vi "Begin.vi"() -> (0 "error out":errorcluster)   [LabVIEW 2013]
doc: "Called before other user functions, this VI is expected to open initial I/O refnums, load in file data, and do all program initialization. Notice that the <B>error out</B> terminal is simply used for data flow. Wiring it to other structures or subVIs ensures that this VI runs first."
uses:
  <vilib>/Rock Robotics/WPI/Joystick/WPI_JoystickDeviceEnum.ctl
  <vilib>/Rock Robotics/SystemInterfaces/Typedef/FPGA_TypedefDigitalModule.ctl
  <vilib>/Rock Robotics/SystemInterfaces/DIO/FPGA_DIOChannel.ctl
  <vilib>/Rock Robotics/SystemInterfaces/DIO/FPGA_DIORelayChannel.ctl
  <vilib>/Rock Robotics/SystemInterfaces/Typedef/FPGA_TypedefSolenoidModule.ctl
  <vilib>/Rock Robotics/WPI/Solenoid/WPI_SolenoidChannel.ctl
  <vilib>/Rock Robotics/WPI/Solenoid/WPI_SolenoidValue.ctl
  <vilib>/Rock Robotics/SystemInterfaces/DIO/FPGA_DIOPWMChannel.ctl
  <vilib>/Rock Robotics/WPI/Encoder/WPI_EncoderType.ctl
  <vilib>/Rock Robotics/WPI/Solenoid/WPI_SolenoidOpenDouble.vi
  <vilib>/Rock Robotics/WPI/Solenoid/WPI_SolenoidSetEnum.vi
  <vilib>/Rock Robotics/WPI/Counter/WPI_CounterDigitalInputToDigitalSource.vi
  <vilib>/Rock Robotics/WPI/RobotDrive/WPI_RobotDriveOpen2MotorWithVictor.vi
  <vilib>/Rock Robotics/WPI/MotorControl/WPI_MotorControlOpen Victor.vi
  <vilib>/Rock Robotics/WPI/Compressor/WPI_CompressorGetSetRefNum.vi
  <vilib>/Rock Robotics/WPI/Camera/WPI_CameraImageSize.ctl
  <vilib>/Rock Robotics/WPI/Camera/WPI_CameraWhite Balance Values.ctl
  <vilib>/Rock Robotics/WPI/Camera/WPI_CameraExposure Values.ctl
  <vilib>/Rock Robotics/WPI/Camera/WPI_CameraFrameRate.ctl
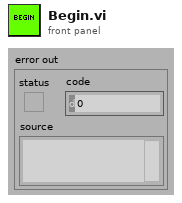
[diagram p1: front panel]
types:
  T1 = typedef "FPGA_DIOChannel.ctl" = enum8{"DIO 1", "DIO 2", "DIO 3", "DIO 4", "DIO 5", "DIO 6", "DIO 7", "DIO 8", "DIO 9", "DIO 10", "DIO 11", "DIO 12", "DIO 13", "DIO 14", "Invalid"}
  T2 = typedef "WPI_SolenoidChannel.ctl" = enum8{"Solenoid 1", "Solenoid 2", "Solenoid 3", "Solenoid 4", "Solenoid 5", "Solenoid 6", "Solenoid 7", "Solenoid 8", "Invalid"}
  T3 = typedef "FPGA_DIOPWMChannel.ctl" = enum8{"PWM 1", "PWM 2", "PWM 3", "PWM 4", "PWM 5", "PWM 6", "PWM 7", "PWM 8", "PWM 9", "PWM 10", "Invalid"}
  T4 = typedef "WPI_EncoderType.ctl" = enum16{"1x", "2x", "4x"}
  T5 = typedef "WPI_SolenoidValue.ctl" = enum16{"Off", "On", "Forward", "Reverse"}
  T6 = typedef "FPGA_TypedefSolenoidModule.ctl" = enum16{"Solenoid Module 1", "Solenoid Module 2"}
  T7 = typedef "FPGA_DIORelayChannel.ctl" = enum8{"Relay 1", "Relay 2", "Relay 3", "Relay 4", "Relay 5", "Relay 6", "Relay 7", "Relay 8", "Invalid"}
  T8 = typedef "WPI_JoystickDeviceEnum.ctl" = enum16{"USB 1", "USB 2", "USB 3", "USB 4", "Kinect 1", "Kinect 2"}
  T9 = typedef "FPGA_TypedefDigitalModule.ctl" = enum16{"Digital Module 1", "Digital Module 2"}
  T10 = typedef "WPI_CameraFrameRate.ctl" = u32
  T11 = typedef "WPI_CameraExposure Values.ctl" = enum16{"Auto", "Flicker-free 50 Hz", "Flicker-free 60 Hz", "Hold current"}
  T12 = typedef "WPI_CameraWhite Balance Values.ctl" = enum16{"Auto", "Fixed indoor", "Fixed outdoor 1", "Fixed outdoor 2", "Fixed fluorescent 1", "Fixed fluorescent 2", "Hold current"}
  T13 = typedef "WPI_CameraImageSize.ctl" = enum16{"640x480", "320x240", "160x120"}
  T14 = typedef "WPI_CameraDevRef.ctl" = cluster{"Camera Address":string, "CameraStatus":errorcluster, "Acquire Image Notifier":refnum<notifier>}
  T15 = typedef "WPI_DigitalInputDevRef.ctl" = cluster{"DevStatus":errorcluster, "DIO Channel":T1, "Digital Module":T9}
  T16 = typedef "WPI_MotorControlDeviceRef.ctl" = cluster{"DeviceStatus":errorcluster, "Type":enum16{"PWM", "CAN"}, "PWM":cluster{"Digital Module":T9, "PWM Channel":T3, "DeadBand":T17}, "CAN":cluster{"Device Number":u8, "Control Mode":T18, "Semaphore":T19, "Max Vout":dbl}, "Invert":bool, "TransformRef":T20, "InvTransformRef":T20}
  T17 = typedef "WPI_PWMDeadband.ctl" = cluster{"Name":string, "maxPositivePwm":i32, "minPositivePwm":i32, "centerPwm":i32, "maxNegativePwm":i32, "minNegativePwm":i32, "angularRange":u16}
  T18 = typedef "WPI_CANJaguar_ControlMode.ctl" = enum8{"Percent VBus", "Current", "Speed", "Position", "Voltage"}
  T19 = typedef "Semaphore RefNum" = refnum<k1>
  T20 = typedef "WPI_PWMTransform_ConPane.ctl" = refnum<vi>
  T21 = typedef "WPI_SolenoidDevRef.ctl" = cluster{"DevStatus":errorcluster, "Solenoid Module":T6, "Forward Solenoid Channel":T2, "Reverse Solenoid Channel":T2}
  T22 = typedef "FPGA_CounterEncoderSourceConvertionLVSourceType.ctl" = cluster{"DevStatus":errorcluster, "AnalogTriggerMode?":bool, "DigitalMode":cluster{"Digital Module":T9, "DIO Channel":T23}, "AnalogTriggerMode":cluster{"AnalogTriggerIndex":T24, "OutputType":T25}}
  T23 = typedef "FPGA_DIODigitalSourceChannel.ctl" = enum8{"DIO 1", "DIO 2", "DIO 3", "DIO 4", "DIO 5", "DIO 6", "DIO 7", "DIO 8", "DIO 9", "DIO 10", "DIO 11", "DIO 12", "DIO 13", "DIO 14", "Disabled"}
  T24 = typedef "FPGA_AnalogTriggerIndex.ctl" = enum8{"Trig 0", "Trig 1", "Trig 2", "Trig 3", "Trig 4", "Trig 5", "Trig 6", "Trig 7", "Invalid"}
  T25 = typedef "FPGA_AnalogTriggerOutType.ctl" = enum16{"InWindow", "TriggerState", "Rising", "Falling"}
  T26 = typedef "WPI_CompressorDevRef.ctl" = cluster{"DevStatus":errorcluster, "DigitalInputDevRef":T15, "RelayDevRef":T27}
  T27 = typedef "WPI_RelayDevRef.ctl" = cluster{"DevStatus":errorcluster, "Relay Channel":T7, "Digital Module":T9, "Relay Direction":T28}
  T28 = typedef "WPI_RelayDirection.ctl" = enum16{"Both directions", "Forward only", "Reverse only"}
  T29 = typedef "WPI_RobotDriveDevRef.ctl" = cluster{"DevStatus":errorcluster, "Motors[]":T16[], "Square Inputs":bool, "Max Output":dbl, "Isochronous":bool}
  T30 = typedef "WPI_EncoderDevRef.ctl" = cluster{"DevStatus":errorcluster, "EncoderIndex":T31, "CounterIndex":T32, "DistancePerCount":dbl, "Decoding Type":T4}
  T31 = typedef "FPGA_EncoderIdx.ctl" = enum8{"Enc 0", "Enc 1", "Enc 2", "Enc 3", "Invalid"}
  T32 = typedef "FPGA_CounterCtrSystemIndex.ctl" = enum8{"Ctr 0", "Ctr 1", "Ctr 2", "Ctr 3", "Ctr 4", "Ctr 5", "Ctr 6", "Ctr 7", "Invalid"}
  T33 = typedef "WPI_JoystickDevRef.ctl" = cluster{"Device":T8}
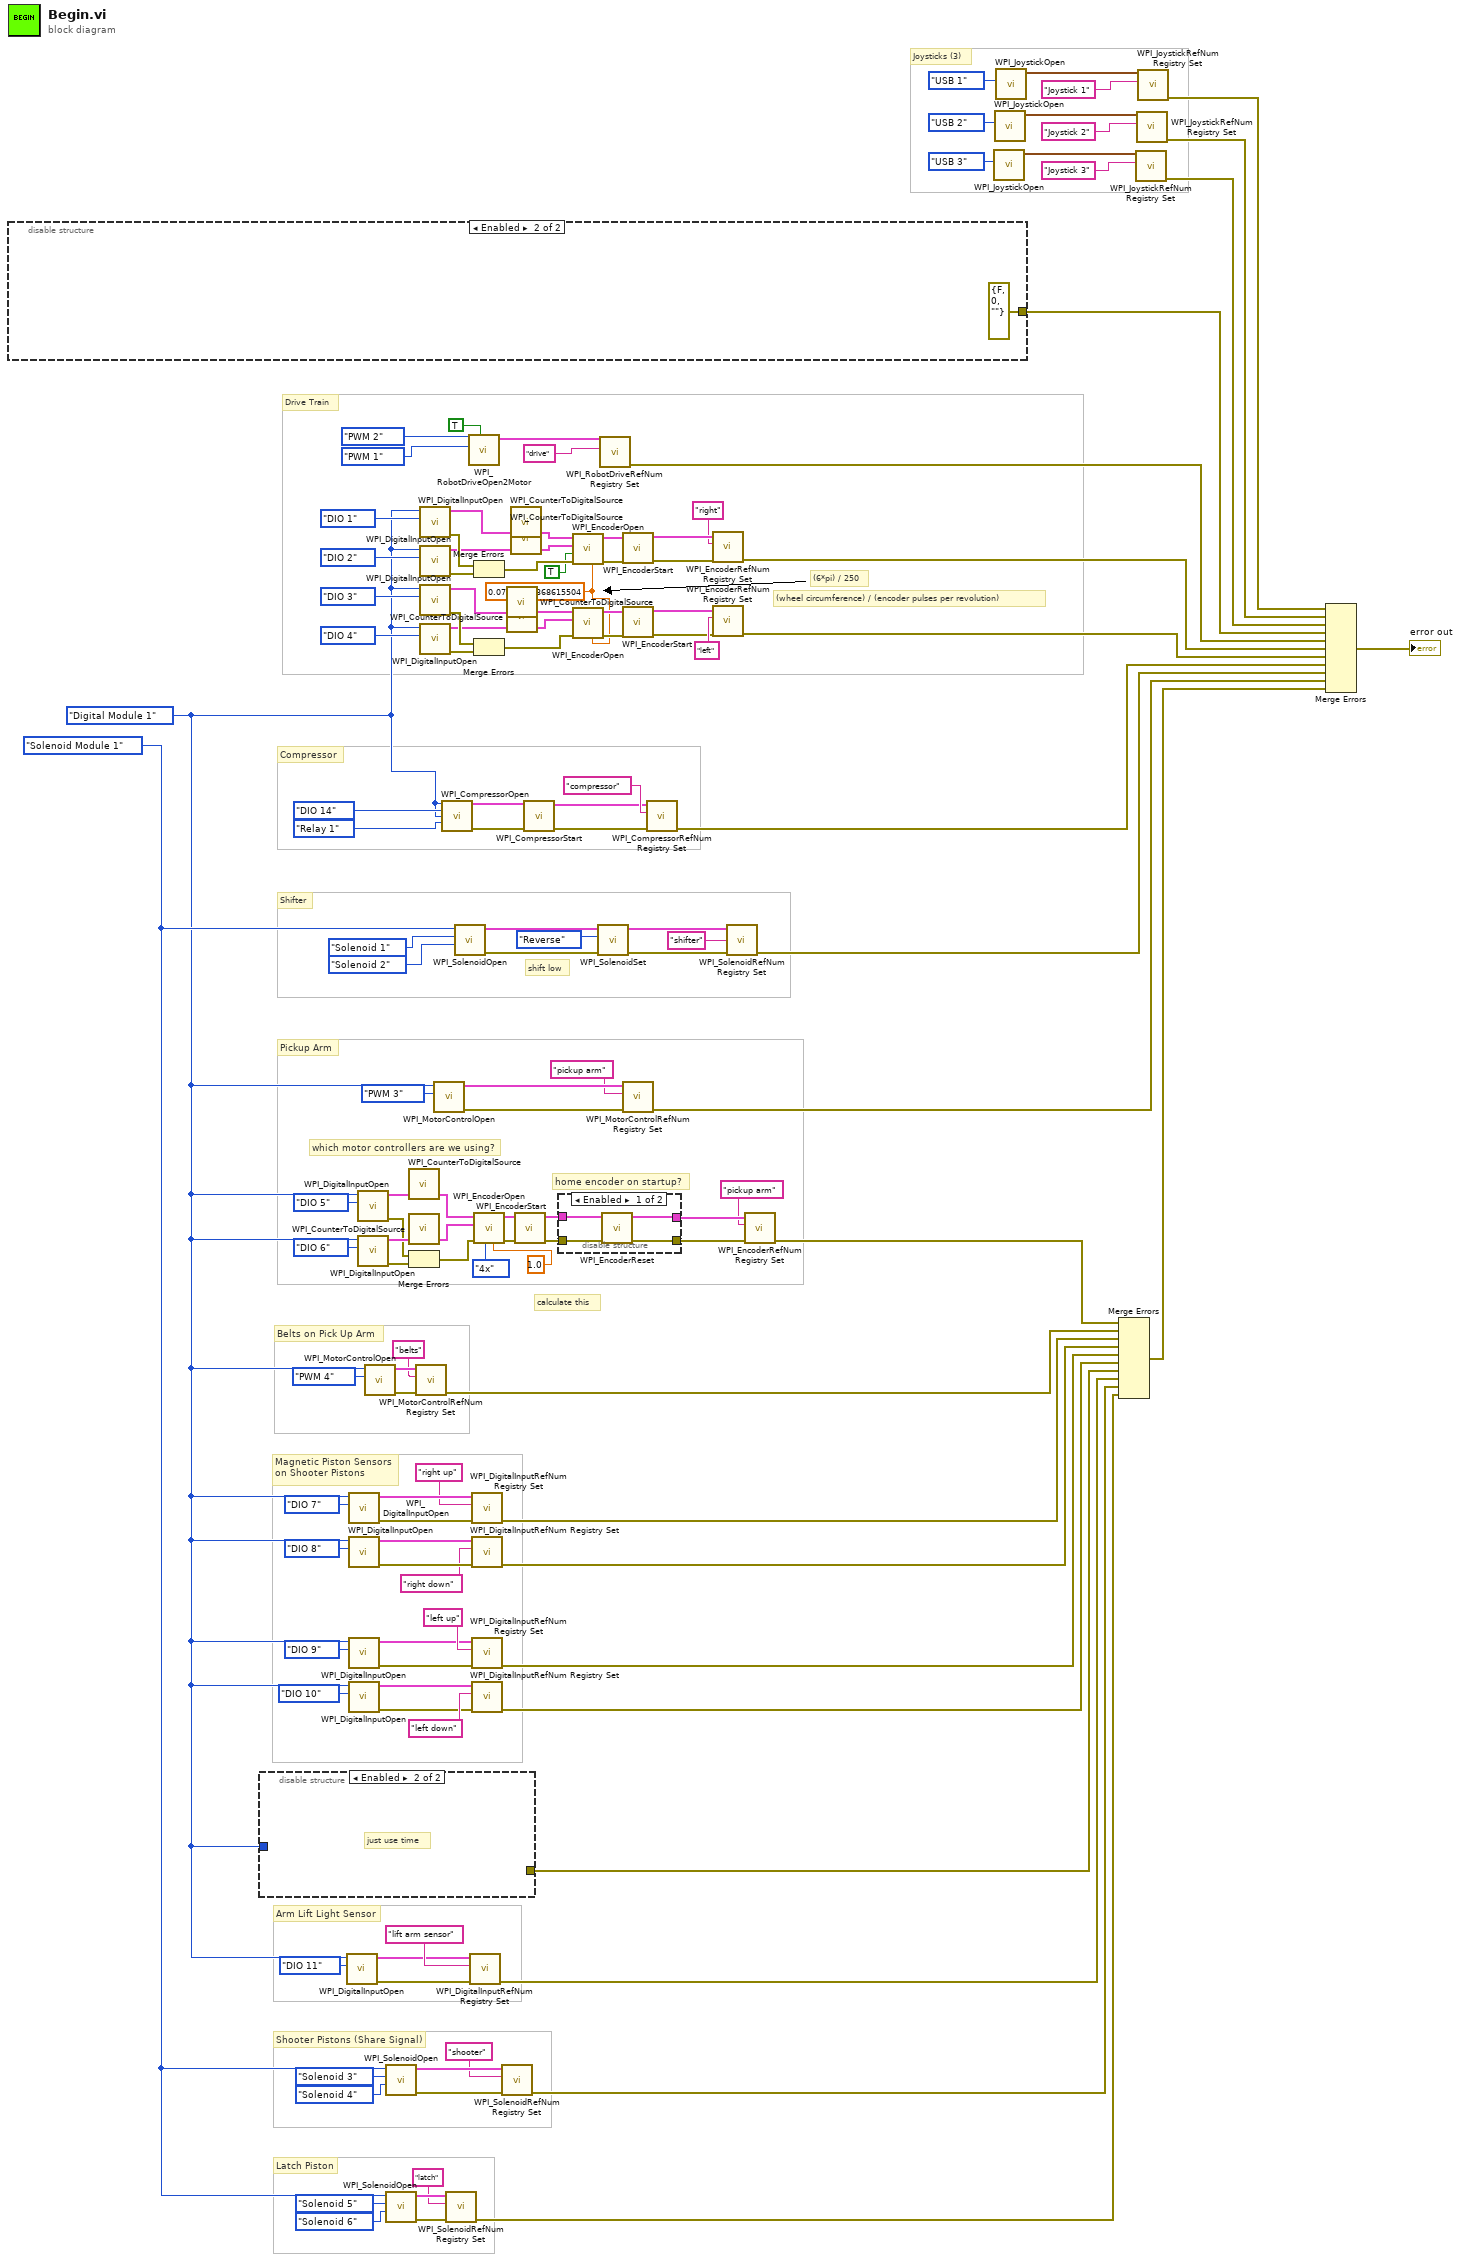
[diagram p0: block diagram]
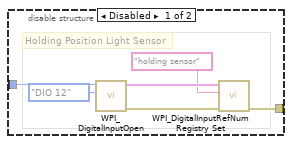
[diagram p2: hidden frame]
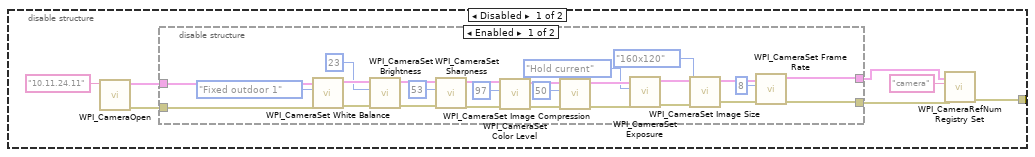
[diagram p4: hidden frame]
diagram:
  w83 = 0.07539822368615504 ("DistancePerCount")
  w20 = FPGA_TypedefSolenoidModule."Solenoid Module 1" ("Solenoid Module (Module 1)")
  w7 = FPGA_TypedefDigitalModule."Digital Module 1" ("Digital Module (Module 1)")
  # "Arm Lift Light Sensor"
  # "Joysticks (3)"
  # "Latch Piston"
  # "Shooter Pistons (Share Signal)"
  # "Magnetic Piston Sensors\non Shooter Pistons"
  # "Belts on Pick Up Arm"
  # "calculate this"
  # "Pickup Arm"
  # "home encoder on startup?"
  # "Shifter"
  # "Compressor"
  # "Drive Train"
  # "which motor controllers are we using?"
  # "shift low"
  # "(wheel circumference) / (encoder pulses per revolution)"
  # "(6*pi) / 250"
  n1 = disable-structure shown="Enabled" {
    disable-tunnel: [w140 errorcluster {"status"=FALSE, "code"=0, "source"=""} ("error out")] -> w127
    frame Disabled {
      n2 = call <vilib>:"WPI_CameraOpen.vi"("Camera Address"="10.11.24.11") -> ("error out"=w142:errorcluster, "CameraDevRef"=w144:T14)  [unwired: 9 in]
      n3 = disable-structure shown="Enabled" {
        disable-tunnel: w144 -> [w170 w174]
        disable-tunnel: [w148 w174] -> w143
        disable-tunnel: w142 -> [w157 w173]
        disable-tunnel: [w147 w173] -> w141
        frame Enabled {
          n4 = call <vilib>:"WPI_CameraSet White Balance.vi"("error in (no error)"=w157, "White Balance"=WPI_CameraWhite_Balance_Values."Fixed outdoor 1", "CameraDevRef"=w170) -> ("error out"=w158:errorcluster, "CameraDevRef Out"=w169:T14)  [unwired: 7 in]
          n5 = call <vilib>:"WPI_CameraSet Brightness.vi"("error in (no error)"=w158, "Brightness"=23, "CameraDevRef"=w169) -> ("error out"=w159:errorcluster, "CameraDevRef Out"=w168:T14)  [unwired: 7 in]
          n6 = call <vilib>:"WPI_CameraSet Sharpness.vi"("error in (no error)"=w159, "Sharpness"=53, "CameraDevRef"=w168) -> ("error out"=w160:errorcluster, "CameraDevRef Out"=w167:T14)  [unwired: 7 in]
          n7 = call <vilib>:"WPI_CameraSet Color Level.vi"("error in (no error)"=w160, "Color Level"=97, "CameraDevRef"=w167) -> ("error out"=w161:errorcluster, "CameraDevRef Out"=w166:T14)  [unwired: 7 in]
          n8 = call <vilib>:"WPI_CameraSet Image Compression.vi"("error in (no error)"=w161, "Compression"=50, "CameraDevRef"=w166) -> ("error out"=w172:errorcluster, "CameraDevRef Out"=w171:T14)  [unwired: 7 in]
          n9 = call <vilib>:"WPI_CameraSet Exposure.vi"("error in (no error)"=w172, "Exposure"=WPI_CameraExposure_Values."Hold current", "CameraDevRef"=w171) -> ("error out"=w162:errorcluster, "CameraDevRef Out"=w165:T14)  [unwired: 7 in]
          n10 = call <vilib>:"WPI_CameraSet Image Size.vi"("error in (no error)"=w162, "Image Size"=WPI_CameraImageSize."160x120", "CameraDevRef"=w165) -> ("error out"=w163:errorcluster, "CameraDevRef Out"=w164:T14)  [unwired: 7 in]
          n11 = call <vilib>:"WPI_CameraSet Frame Rate.vi"("error in (no error)"=w163, "Frame Rate (fps)"=T10 8, "CameraDevRef"=w164) -> ("error out"=w147:errorcluster, "CameraDevRef Out"=w148:T14)  [unwired: 7 in]
        }
        frame Disabled {
        }
      }
      n12 = call <vilib>:"WPI_CameraRefNum Registry Set.vi"("error in (no error)"=w141, "refnum name"="camera", "CameraDevRef"=w143) -> ("error out"=w140:errorcluster)  [unwired: 7 in, 1 out]
    }
    frame Enabled {
    }
  }
  n13 = disable-structure shown="Enabled" {
    disable-tunnel: w7 -> [w177 _]
    disable-tunnel: [w176 _] -> w3
    frame Disabled {
      # "Holding Position Light Sensor"
      n14 = call <vilib>:"WPI_DigitalInputOpen.vi"("DIO Channel"=FPGA_DIOChannel."DIO 12", "Digital Module (Module 1)"=w177) -> ("error out"=w180:errorcluster, "DigitalInputDevRef"=w179:T15)  [unwired: 8 in]
      n15 = call <vilib>:"WPI_DigitalInputRefNum Registry Set.vi"("error in (no error)"=w180, "refnum name"="holding sensor", "DigitalInputDevRef"=w179) -> ("error out"=w176:errorcluster)  [unwired: 7 in, 1 out]
    }
    frame Enabled {
      # "just use time"
    }
  }
  n16 = call <vilib>:"WPI_DigitalInputOpen.vi"("DIO Channel"=FPGA_DIOChannel."DIO 11", "Digital Module (Module 1)"=w7) -> ("error out"=w17:errorcluster, "DigitalInputDevRef"=w18:T15)  [unwired: 8 in]
  n17 = call <vilib>:"WPI_DigitalInputOpen.vi"("DIO Channel"=FPGA_DIOChannel."DIO 7", "Digital Module (Module 1)"=w7) -> ("error out"=w40:errorcluster, "DigitalInputDevRef"=w39:T15)  [unwired: 8 in]
  n18 = call <vilib>:"WPI_DigitalInputOpen.vi"("DIO Channel"=FPGA_DIOChannel."DIO 8", "Digital Module (Module 1)"=w7) -> ("error out"=w38:errorcluster, "DigitalInputDevRef"=w37:T15)  [unwired: 8 in]
  n19 = call <vilib>:"WPI_DigitalInputOpen.vi"("DIO Channel"=FPGA_DIOChannel."DIO 9", "Digital Module (Module 1)"=w7) -> ("error out"=w8:errorcluster, "DigitalInputDevRef"=w9:T15)  [unwired: 8 in]
  n20 = call <vilib>:"WPI_DigitalInputOpen.vi"("DIO Channel"=FPGA_DIOChannel."DIO 10", "Digital Module (Module 1)"=w7) -> ("error out"=w10:errorcluster, "DigitalInputDevRef"=w11:T15)  [unwired: 8 in]
  n21 = call <vilib>:"WPI_DigitalInputOpen.vi"("DIO Channel"=FPGA_DIOChannel."DIO 5", "Digital Module (Module 1)"=w7) -> ("error out"=w58:errorcluster, "DigitalInputDevRef"=w63:T15)  [unwired: 8 in]
  n22 = call <vilib>:"WPI_DigitalInputOpen.vi"("DIO Channel"=FPGA_DIOChannel."DIO 6", "Digital Module (Module 1)"=w7) -> ("error out"=w59:errorcluster, "DigitalInputDevRef"=w62:T15)  [unwired: 8 in]
  n23 = call-poly <vilib>:"WPI_MotorControlOpen.vi"("PWM Channel"=FPGA_DIOPWMChannel."PWM 4", "Digital Module (Module 1)"=w7) -> ("error out"=w46:errorcluster, "MotorControlDeviceRef"=w45:T16)  [unwired: 8 in]
  n24 = call-poly <vilib>:"WPI_SolenoidOpen.vi"("Reverse Solenoid Channel"=WPI_SolenoidChannel."Solenoid 4", "Forward Solenoid Channel"=WPI_SolenoidChannel."Solenoid 3", "Solenoid Module (Module 1)"=w20) -> ("error out"=w26:errorcluster, "SolenoidDevRef"=w25:T21)  [unwired: 7 in]
  n25 = call-poly <vilib>:"WPI_SolenoidOpen.vi"("Reverse Solenoid Channel"=WPI_SolenoidChannel."Solenoid 6", "Forward Solenoid Channel"=WPI_SolenoidChannel."Solenoid 5", "Solenoid Module (Module 1)"=w20) -> ("error out"=w24:errorcluster, "SolenoidDevRef"=w23:T21)  [unwired: 7 in]
  n26 = call-poly <vilib>:"WPI_CounterToDigitalSource.vi"("DigitalInputDevRef"=w63) -> ("Digital Source"=w61:T22)  [unwired: 6 in]
  n27 = call-poly <vilib>:"WPI_CounterToDigitalSource.vi"("DigitalInputDevRef"=w62) -> ("Digital Source"=w60:T22)  [unwired: 6 in]
  n28 = Merge Errors(w58, w59) -> (w57:errorcluster)
  n29 = call <vilib>:"WPI_MotorControlRefNum Registry Set.vi"("error in (no error)"=w46, "refnum name"="belts", "MotorControlDevRef"=w45) -> ("error out"=w43:errorcluster)  [unwired: 7 in, 1 out]
  n30 = call <vilib>:"WPI_DigitalInputOpen.vi"("DIO Channel"=FPGA_DIOChannel."DIO 1", "Digital Module (Module 1)"=w7) -> ("error out"=w77:errorcluster, "DigitalInputDevRef"=w91:T15)  [unwired: 8 in]
  n31 = call <vilib>:"WPI_DigitalInputOpen.vi"("DIO Channel"=FPGA_DIOChannel."DIO 2", "Digital Module (Module 1)"=w7) -> ("error out"=w79:errorcluster, "DigitalInputDevRef"=w76:T15)  [unwired: 8 in]
  n32 = call <vilib>:"WPI_DigitalInputOpen.vi"("DIO Channel"=FPGA_DIOChannel."DIO 3", "Digital Module (Module 1)"=w7) -> ("error out"=w80:errorcluster, "DigitalInputDevRef"=w105:T15)  [unwired: 8 in]
  n33 = call <vilib>:"WPI_DigitalInputOpen.vi"("DIO Channel"=FPGA_DIOChannel."DIO 4", "Digital Module (Module 1)"=w7) -> ("error out"=w82:errorcluster, "DigitalInputDevRef"=w75:T15)  [unwired: 8 in]
  n34 = call-poly <vilib>:"WPI_MotorControlOpen.vi"("PWM Channel"=FPGA_DIOPWMChannel."PWM 3", "Digital Module (Module 1)"=w7) -> ("error out"=w70:errorcluster, "MotorControlDeviceRef"=w69:T16)  [unwired: 8 in]
  n35 = call <vilib>:"WPI_CompressorOpen.vi"("Pressure Switch Digital Module (Module 1)"=w7, "Pressure Switch DIO Channel"=FPGA_DIOChannel."DIO 14", "Relay Digital Module (Module 1)"=w7, "Relay Channel"=FPGA_DIORelayChannel."Relay 1") -> ("CompressorDevRef"=w119:T26, "error out"=w118:errorcluster)  [unwired: 10 in]
  n36 = call <vilib>:"WPI_SolenoidRefNum Registry Set.vi"("error in (no error)"=w24, "refnum name"="latch", "SolenoidDevRef"=w23) -> ("error out"=w6:errorcluster)  [unwired: 7 in, 1 out]
  n37 = call-poly <vilib>:"WPI_SolenoidOpen.vi"("Reverse Solenoid Channel"=WPI_SolenoidChannel."Solenoid 2", "Forward Solenoid Channel"=WPI_SolenoidChannel."Solenoid 1", "Solenoid Module (Module 1)"=w20) -> ("error out"=w110:errorcluster, "SolenoidDevRef"=w111:T21)  [unwired: 7 in]
  n38 = call-poly <vilib>:"WPI_RobotDriveOpen2Motor.vi"("Left Motor Inverted"=TRUE, "Right Motor"=FPGA_DIOPWMChannel."PWM 1", "Left Motor"=FPGA_DIOPWMChannel."PWM 2") -> ("RobotDriveDevRef"=w107:T29)  [unwired: 7 in, 1 out]
  n39 = call <vilib>:"WPI_DigitalInputRefNum Registry Set.vi"("error in (no error)"=w17, "refnum name"="lift arm sensor", "DigitalInputDevRef"=w18) -> ("error out"=w4:errorcluster)  [unwired: 7 in, 1 out]
  n40 = call <vilib>:"WPI_DigitalInputRefNum Registry Set.vi"("error in (no error)"=w40, "refnum name"="right up", "DigitalInputDevRef"=w39) -> ("error out"=w33:errorcluster)  [unwired: 7 in, 1 out]
  n41 = call <vilib>:"WPI_DigitalInputRefNum Registry Set.vi"("error in (no error)"=w38, "refnum name"="right down", "DigitalInputDevRef"=w37) -> ("error out"=w32:errorcluster)  [unwired: 7 in, 1 out]
  n42 = call <vilib>:"WPI_DigitalInputRefNum Registry Set.vi"("error in (no error)"=w8, "refnum name"="left up", "DigitalInputDevRef"=w9) -> ("error out"=w2:errorcluster)  [unwired: 7 in, 1 out]
  n43 = call <vilib>:"WPI_DigitalInputRefNum Registry Set.vi"("error in (no error)"=w10, "refnum name"="left down", "DigitalInputDevRef"=w11) -> ("error out"=w1:errorcluster)  [unwired: 7 in, 1 out]
  n44 = Merge Errors(w77, w79) -> (w78:errorcluster)
  n45 = Merge Errors(w80, w82) -> (w81:errorcluster)
  n46 = call <vilib>:"WPI_EncoderOpen.vi"("DistancePerCount"=1.0, "Decoding Type"=WPI_EncoderType."4x", "error in (no error)"=w57, "BSource"=w60, "ASource"=w61) -> ("error out"=w56:errorcluster, "EncoderDevRef"=w55:T30)  [unwired: 5 in]
  n47 = call <vilib>:"WPI_SolenoidRefNum Registry Set.vi"("error in (no error)"=w26, "refnum name"="shooter", "SolenoidDevRef"=w25) -> ("error out"=w5:errorcluster)  [unwired: 7 in, 1 out]
  n48 = call-poly <vilib>:"WPI_CounterToDigitalSource.vi"("DigitalInputDevRef"=w105) -> ("Digital Source"=w98:T22)  [unwired: 6 in]
  n49 = call-poly <vilib>:"WPI_CounterToDigitalSource.vi"("DigitalInputDevRef"=w75) -> ("Digital Source"=w99:T22)  [unwired: 6 in]
  n50 = call-poly <vilib>:"WPI_CounterToDigitalSource.vi"("DigitalInputDevRef"=w91) -> ("Digital Source"=w97:T22)  [unwired: 6 in]
  n51 = call-poly <vilib>:"WPI_CounterToDigitalSource.vi"("DigitalInputDevRef"=w76) -> ("Digital Source"=w96:T22)  [unwired: 6 in]
  n52 = call <vilib>:"WPI_EncoderStart.vi"("error in (no error)"=w56, "EncoderDevRef"=w55) -> ("error out"=w54:errorcluster, "EncoderDevRef"=w53:T30)  [unwired: 8 in]
  n53 = call <vilib>:"WPI_CompressorStart.vi"("error in (no error)"=w118, "CompressorDevRef"=w119) -> ("error out"=w117:errorcluster, "CompressorDevRef"=w116:T26)  [unwired: 8 in]
  n54 = disable-structure shown="Enabled" {
    disable-tunnel: w54 -> [w185 w186]
    disable-tunnel: w53 -> [w184 w187]
    disable-tunnel: [w183 w187] -> w51
    disable-tunnel: [w182 w186] -> w52
    frame Enabled {
      n55 = call <vilib>:"WPI_EncoderReset.vi"("error in (no error)"=w185, "EncoderDevRef"=w184) -> ("error out"=w182:errorcluster, "EncoderDevRef"=w183:T30)  [unwired: 8 in]
    }
    frame Disabled {
    }
  }
  n56 = call <vilib>:"WPI_EncoderOpen.vi"("DistancePerCount"=w83, "error in (no error)"=w78, "Invert Direction (False)"=TRUE, "BSource"=w96, "ASource"=w97) -> ("error out"=w95:errorcluster, "EncoderDevRef"=w94:T30)  [unwired: 5 in]
  n57 = call <vilib>:"WPI_EncoderOpen.vi"("DistancePerCount"=w83, "error in (no error)"=w81, "BSource"=w99, "ASource"=w98) -> ("error out"=w100:errorcluster, "EncoderDevRef"=w101:T30)  [unwired: 6 in]
  n58 = call-poly <vilib>:"WPI_SolenoidSet.vi"("error in (no error)"=w110, "Value"=WPI_SolenoidValue."Reverse", "SolenoidDevRef"=w111) -> ("error out"=w109:errorcluster, "SolenoidDevRef"=w108:T21)  [unwired: 7 in]
  n59 = call <vilib>:"WPI_RobotDriveRefNum Registry Set.vi"("refnum name"="drive", "RobotDriveDevRef"=w107) -> ("error out"=w126:errorcluster)  [unwired: 8 in, 1 out]
  n60 = call <vilib>:"WPI_EncoderStart.vi"("error in (no error)"=w95, "EncoderDevRef"=w94) -> ("error out"=w93:errorcluster, "EncoderDevRef"=w92:T30)  [unwired: 8 in]
  n61 = call <vilib>:"WPI_EncoderStart.vi"("error in (no error)"=w100, "EncoderDevRef"=w101) -> ("error out"=w102:errorcluster, "EncoderDevRef"=w103:T30)  [unwired: 8 in]
  n62 = call <vilib>:"WPI_MotorControlRefNum Registry Set.vi"("error in (no error)"=w70, "refnum name"="pickup arm", "MotorControlDevRef"=w69) -> ("error out"=w66:errorcluster)  [unwired: 7 in, 1 out]
  n63 = call <vilib>:"WPI_CompressorRefNum Registry Set.vi"("error in (no error)"=w117, "refnum name"="compressor", "CompressorDevRef"=w116) -> ("error out"=w71:errorcluster)  [unwired: 7 in, 1 out]
  n64 = call <vilib>:"WPI_EncoderRefNum Registry Set.vi"("error in (no error)"=w93, "refnum name"="right", "EncoderDevRef"=w92) -> ("error out"=w125:errorcluster)  [unwired: 7 in, 1 out]
  n65 = call <vilib>:"WPI_EncoderRefNum Registry Set.vi"("error in (no error)"=w102, "refnum name"="left", "EncoderDevRef"=w103) -> ("error out"=w124:errorcluster)  [unwired: 7 in, 1 out]
  n66 = call <vilib>:"WPI_SolenoidRefNum Registry Set.vi"("error in (no error)"=w109, "refnum name"="shifter", "SolenoidDevRef"=w108) -> ("error out"=w72:errorcluster)  [unwired: 7 in, 1 out]
  n67 = call <vilib>:"WPI_EncoderRefNum Registry Set.vi"("error in (no error)"=w52, "refnum name"="pickup arm", "EncoderDevRef"=w51) -> ("error out"=w42:errorcluster)  [unwired: 7 in, 1 out]
  n68 = call <vilib>:"WPI_JoystickOpen.vi"("JoystickDevice"=WPI_JoystickDeviceEnum."USB 3") -> ("JoystickDevRef"=w138:T33)  [unwired: 10 in]
  n69 = call <vilib>:"WPI_JoystickOpen.vi"("JoystickDevice"=WPI_JoystickDeviceEnum."USB 2") -> ("JoystickDevRef"=w135:T33)  [unwired: 10 in]
  n70 = call <vilib>:"WPI_JoystickOpen.vi"("JoystickDevice"=WPI_JoystickDeviceEnum."USB 1") -> ("JoystickDevRef"=w132:T33)  [unwired: 10 in]
  n71 = Merge Errors(w42, w43, w33, w32, w2, w1, w3, w4, w5, w6) -> (w41:errorcluster)
  n72 = call <vilib>:"WPI_JoystickRefNum Registry Set.vi"("refnum name"="Joystick 3", "JoystickDevRef"=w138) -> ("error out"=w128:errorcluster)  [unwired: 8 in, 1 out]
  n73 = call <vilib>:"WPI_JoystickRefNum Registry Set.vi"("refnum name"="Joystick 2", "JoystickDevRef"=w135) -> ("error out"=w129:errorcluster)  [unwired: 8 in, 1 out]
  n74 = call <vilib>:"WPI_JoystickRefNum Registry Set.vi"("refnum name"="Joystick 1", "JoystickDevRef"=w132) -> ("error out"=w130:errorcluster)  [unwired: 8 in, 1 out]
  n75 = Merge Errors(w130, w129, w128, w127, w126, w125, w124, w71, w72, w66, w41) -> (→"error out":errorcluster)
